vi "CountTime.vi"() -> ()   [LabVIEW 2018]
panel:
  in  "?":bool
  out "Hours":dbl
  out "Minutes":dbl
  out "Seconds":dbl
  in  "Time In \nSeconds":dbl
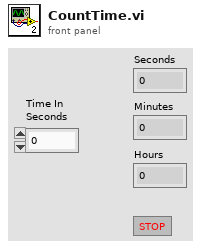
[diagram p1: front panel]
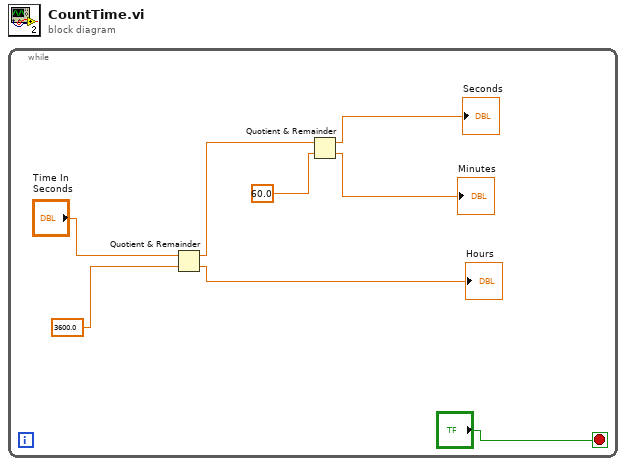
[diagram p0: block diagram]
diagram:
  n1 = while {
    stop <- "?" stop-if-true
    n2 = Quotient & Remainder(x="Time In \nSeconds", y=3600.0) -> (x-y*floor(x/y)=w5:dbl, floor(x/y)=→"Hours":dbl)
    n3 = Quotient & Remainder(x=w5, y=60.0) -> (x-y*floor(x/y)=→"Seconds":dbl, floor(x/y)=→"Minutes":dbl)
  }
